vi "Log User Event.vi"(8 "error in (no error)":errorcluster, 11 "S4GUI in":refnum<class "S4GUI.lvclass">) -> (0 "error out":errorcluster, 3 "S4GUI out":refnum<class "S4GUI.lvclass">)   [LabVIEW 2018, in "S4GUI.lvclass"]
uses:
  S4GUI.lvclass
  S4GUI.lvclass/S4GUI.ctl
  Log/Log.lvclass
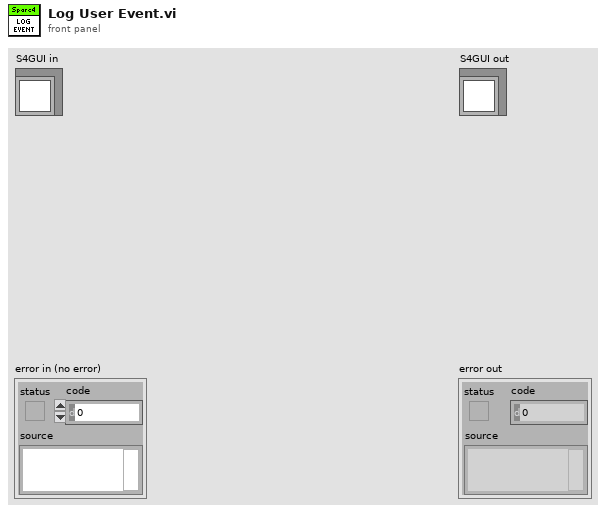
[diagram p1: front panel]
types:
  T1 = enum16{"INFO ", "TRACE", "DEBUG", "WARN ", "ERROR", "FATAL", "OTHER"}
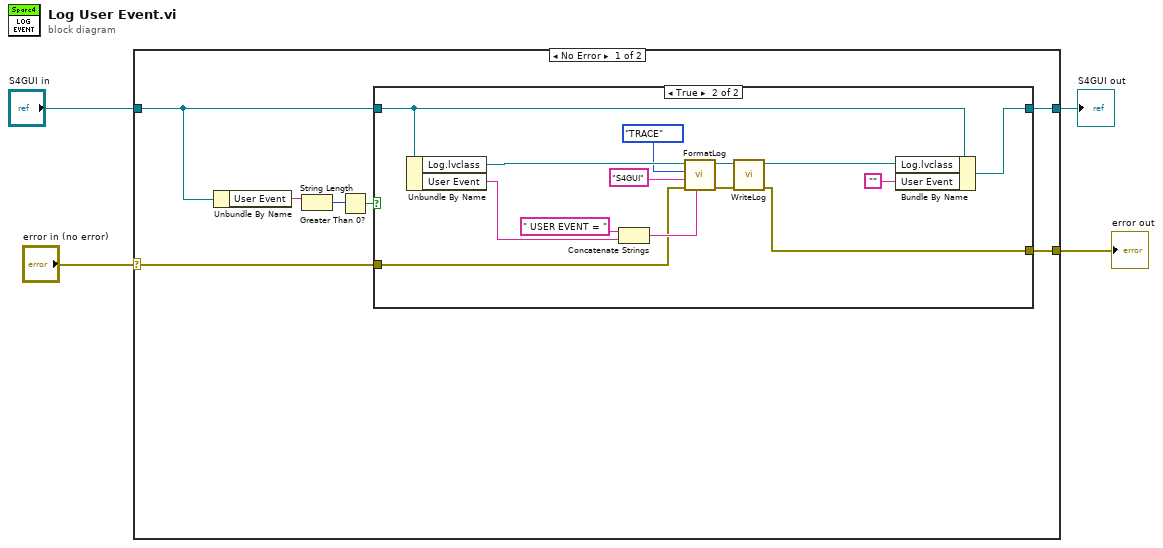
[diagram p0: block diagram]
diagram:
  n1 = case shown="No Error" "error in (no error)" {
    selector: "error in (no error)" -> [w6 w29]
    tunnel: [w5 w29] -> w3
    tunnel: [w7 w28] -> w1
    tunnel: "S4GUI in" -> [w8 w28]
    frame No Error {
      n2 = Unbundle By Name(w8) -> ("User Event"=w11:string)
      n3 = String Length(string=w11) -> (length=w10:i32)
      n4 = Greater Than 0?(x=w10) -> (x > 0?=w9:bool)
      n5 = case shown="True" w9 {
        tunnel: w8 -> [w13 w27]
        tunnel: [w13 w26] -> w7
        tunnel: w6 -> [w12 w18]
        tunnel: [w12 w15] -> w5
        frame False {
        }
        frame True {
          n6 = Unbundle By Name(w27) -> ("Log.lvclass"=w17:refnum<class "Log.lvclass">, "User Event"=w19:string)
          n7 = Concatenate Strings(" USER EVENT = " ("string"), w19) -> (w20:string)
          n8 = call-dynamic "FormatLog.vi"("log input"=w20, "error in (no error)"=w18, "System"="S4GUI", "Type"=T1."TRACE", "Log in"=w17) -> ("error out"=w23:errorcluster, "Log out"=w24:refnum<class "Log.lvclass">)  [unwired: 5 in]
          n9 = call-dynamic "WriteLog.vi"("error in (no error)"=w23, "Log in"=w24) -> ("error out"=w15:errorcluster, "Log out"=w16:refnum<class "Log.lvclass">)  [unwired: 8 in]
          n10 = Bundle By Name(cluster=w27, "Log.lvclass"=w16, "User Event"="") -> (w26:refnum<class "S4GUI.lvclass">)
        }
      }
    }
    frame Error {
    }
  }
  "error out" <- w3
  "S4GUI out" <- w1
